vi "HistogramSaturation.vi"(11 "Histogram Report":T1) -> ()   [LabVIEW 2015]
panel:
  out "ElementNumber":u32
  out "fractional index or x":dbl
  in  "GainVariable 2":u64
  in  "Gain permitted values":u32[](array[numeric])=[0, 16, 32, 48, 64, 80, 96, 112, 128, 144, 160, 176, 192, 208, 224, 240, 256, 288, 320, 352, 384, 416, 448, 480, 512, 544, 576, 608, 640, 672, 704, 736, 768, 832, 896, 960, 1024, 1088, 1152, 1216, 1280, 1344, 1408, 1472, 1536, 1600, 1664, 1728]
  out "x/y":dbl
  out "sum":u32
  out "size(s)":i32
  out "subarray":u32[](array[numeric])
  in  "Max Intensity":dbl=250.0 max=254.0
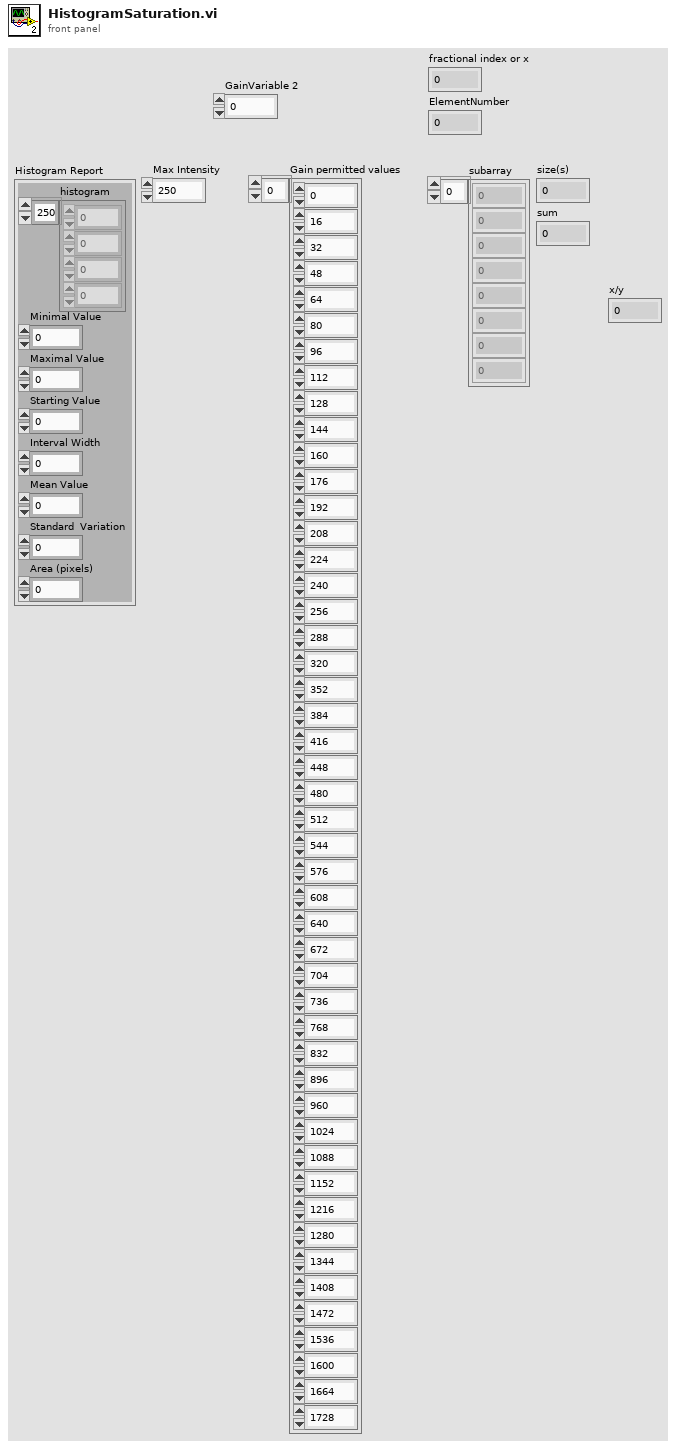
[diagram p1: front panel]
types:
  T1 = cluster{"histogram":u32[], "Minimal Value":sgl, "Maximal Value":sgl, "Starting Value":sgl, "Interval Width":sgl, "Mean Value":sgl, "Standard  Variation":sgl, "Area (pixels)":i32}
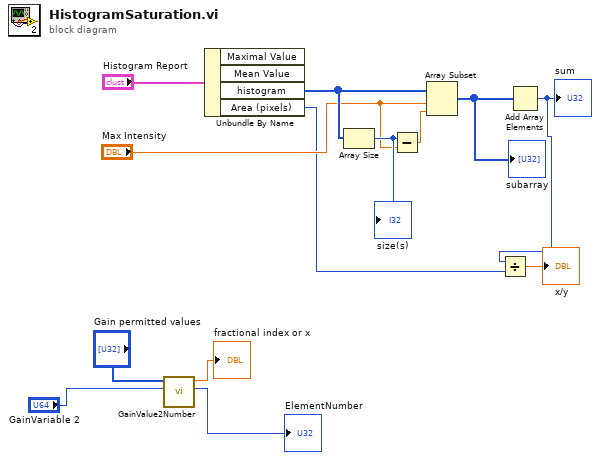
[diagram p0: block diagram]
diagram:
  n1 = call "GainValue2Number.vi"("GainValue"="GainVariable 2", "Gain permitted values"="Gain permitted values") -> ("Value out"=→"ElementNumber":u32, "fractional index or x"=→"fractional index or x":dbl)  [unwired: 8 in]
  n2 = Unbundle By Name("Histogram Report") -> ("histogram"=w12:u32[], "Area (pixels)"=w6:i32)  [unwired: 2 out]
  n3 = Array Size(array=w12) -> (size(s)=w10:i32)
  "size(s)" <- w10
  n4 = Subtract(x=w10, y="Max Intensity") -> (x-y=w11:dbl)
  n5 = Array Subset(array=w12, index="Max Intensity", length=w11) -> (w8:u32[])
  "subarray" <- w8
  n6 = Add Array Elements(numeric array=w8) -> (sum=w7:u32)
  "sum" <- w7
  n7 = Divide(x=w7, y=w6) -> (x/y=→"x/y":dbl)
